vi "Square Input.vi"(1 "Input":dbl) -> (0 "Output Squared":dbl)   [LabVIEW 2020]
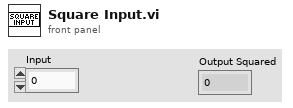
[diagram p1: front panel]
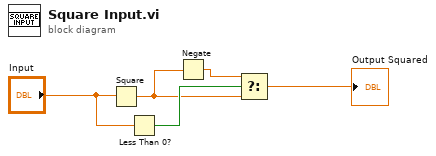
[diagram p0: block diagram]
diagram:
  n1 = Square(x="Input") -> (x^2=w2:dbl)
  n2 = Less Than 0?(x="Input") -> (x < 0?=w3:bool)
  n3 = Negate(x=w2) -> (-x=w1:dbl)
  n4 = Select(t=w1, s=w3, f=w2) -> (s? t:f=→"Output Squared":dbl)
